vi "SaveData.vi"(8 "에러 입력":errorcluster, 9 "Index":i32, 10 "배열":T1(array[cluster]), 11 "참조번호":refnum<file>) -> (0 "에러 출력":errorcluster, 1 "Index 2":i32, 3 "참조 번호 출력":refnum<file>)   [LabVIEW 2019]
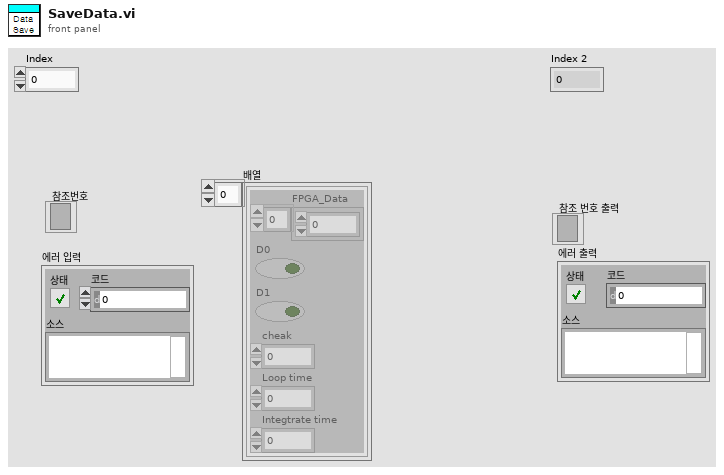
[diagram p1: front panel]
types:
  T1 = cluster{"FPGA_Data":sgl[], "D0":bool, "D1":bool, "cheak":i32, "Loop time":dbl, "Integtrate time":dbl}[]
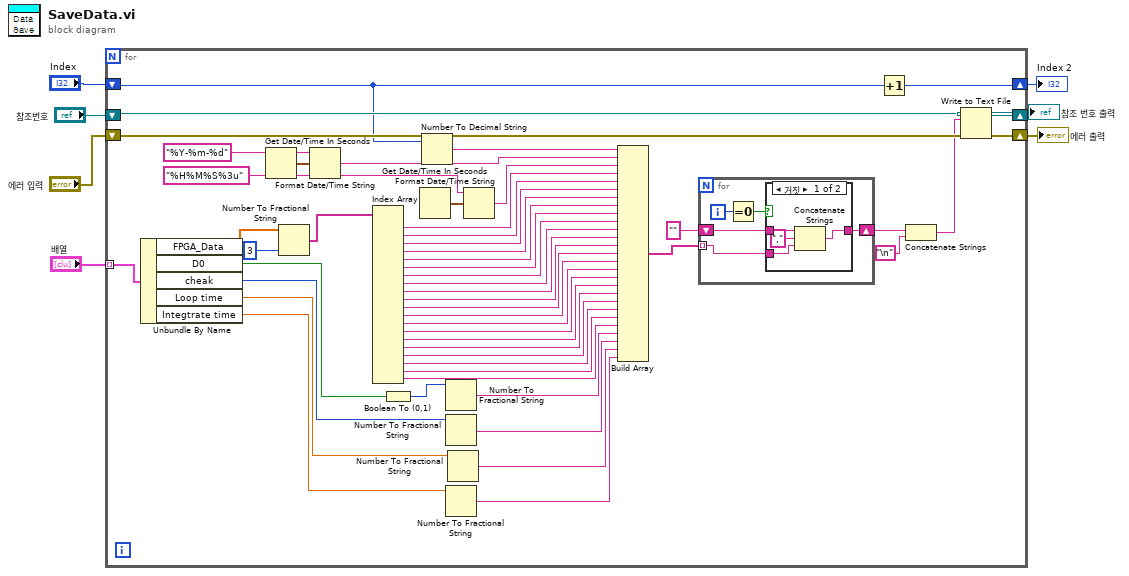
[diagram p0: block diagram]
diagram:
  n1 = for {
    shift-right: [w53] -> w4
    shift-left: "에러 입력" -> [w55]
    shift-right: [w54] -> w5
    shift-left: "참조번호" -> [w20]
    shift-right: [w12] -> w2
    shift-left: "Index" -> [w13]
    tunnel: "배열" -> [w16] mode=indexing
    n2 = Unbundle By Name(w16) -> ("FPGA_Data"=w47:sgl[], "D0"=w49:bool, "cheak"=w45:i32, "Loop time"=w11:dbl, "Integtrate time"=w10:dbl)
    n3 = Get Date/Time In Seconds() -> (seconds since 1Jan1904=w58:timestamp)
    n4 = Number To Fractional String(number=w47, precision (6)=i16 3 ("정밀도(6)")) -> (F-format string=w46:string[])  [unwired: 2 in]
    n5 = Format Date/Time String(time format string (%c)="%Y-%m-%d" ("시간 포맷 문자열 (%c)"), seconds (now)=w58) -> (date/time string=w44:string)  [unwired: 1 in]
    n6 = Index Array(array=w46) -> (element #1=w42:string, element #2=w41:string, element #3=w40:string, element #4=w39:string, element #5=w38:string, element #6=w37:string, element #7=w36:string, element #8=w35:string, element #9=w34:string, element #10=w33:string, element #11=w32:string, element #12=w31:string, element #13=w30:string, element #14=w29:string, element #15=w28:string, element #16=w27:string, element #17=w26:string, element #18=w25:string, element #19=w24:string, element #20=w23:string)  [unwired: 20 in]
    n7 = Boolean To (0,1)(Boolean=w49) -> (0, 1=w48:i16)
    n8 = Get Date/Time In Seconds() -> (seconds since 1Jan1904=w52:timestamp)
    n9 = Number To Decimal String(number=w13) -> (decimal integer string=w56:string)  [unwired: 1 in]
    n10 = Number To Fractional String(number=w48) -> (F-format string=w22:string)  [unwired: 3 in]
    n11 = Number To Fractional String(number=w45) -> (F-format string=w21:string)  [unwired: 3 in]
    n12 = Number To Fractional String(number=w10) -> (F-format string=w8:string)  [unwired: 3 in]
    n13 = Number To Fractional String(number=w11) -> (F-format string=w9:string)  [unwired: 3 in]
    n14 = Format Date/Time String(time format string (%c)="%H%M%S%3u" ("시간 포맷 문자열 (%c)"), seconds (now)=w52) -> (date/time string=w43:string)  [unwired: 1 in]
    n15 = Build Array(w56, w44, w43, w42, w41, w40, w39, w38, w37, w36, w35, w34, w33, w32, w31, w30, w29, w28, w27, w26, w25, w24, w23, w22, w21, w9, w8) -> (w15:string[])
    n16 = for {
      shift-right: [w60] -> w18
      shift-left: "" -> [w61]
      tunnel: w15 -> [w59] mode=indexing
      i -> [w63]
      n17 = Equal To 0?(x=w63) -> (x = 0?=w62:bool)
      n18 = case shown="거짓" w62 {
        tunnel: w61 -> [w67 w68]
        tunnel: [w66 w68] -> w60
        tunnel: w59 -> [w64 _]
        frame False {
          n19 = Concatenate Strings(w67, "," ("문자열"), w64) -> (w66:string)
        }
        frame True {
        }
      }
    }
    n20 = Increment(x=w13) -> (x+1=w12:i32)
    n21 = Concatenate Strings(w18, "\n") -> (w19:string)
    n22 = Write to Text File(file (use dialog)=w20, text=w19, error in=w55) -> (refnum out=w54:refnum<file>, error out=w53:errorcluster)  [unwired: 1 in, 1 out]
  }
  "참조 번호 출력" <- w5
  "에러 출력" <- w4
  "Index 2" <- w2
